vi "Rev_archivos_Calibracion.vi"() -> ()   [LabVIEW 2015]
uses:
  <vilib>/Analysis/3filter.llb/Filter Passband Type.ctl
  <vilib>/Analysis/5stat.llb/RMS (DBL).vi
  <vilib>/Analysis/baseanly.llb/Mean (DBL).vi
  <vilib>/Analysis/3filter.llb/Butterworth Filter (DBL).vi
  <vilib>/measure/madcrms.llb/Basic Averaged DC-RMS for 1 Chan.vi
  <vilib>/measure/maspectr.llb/FFT Spectrum (Mag-Phase) for 1 Chan.vi
  <vilib>/Analysis/NI_AALBase.lvlib
  <vilib>/measure/NI_MAPro.lvlib
  <vilib>/Analysis/NI_AALPro.lvlib
panel:
  out "RMS conseguido":dbl format="%0.2f"
  in  "Frecuencia de excitación\ndel patrón (Hz)":sgl=159.2
  in  "Aceleración del\npatrón (g RMS)":sgl=1.0
  out "% de desv":dbl
  in  "file (use dialog)":path
  in  "Nº del canal":i32
  out "Desviación típica":dbl format="%0.2f"
  out "Promedio":dbl format="%0.2f"
  in  "Parámetro de sensibilidad\n           (mV/g) 2":sgl=10.0
  out "Número de muestras":i32
  out "FFT de la señal":cluster{"f0":dbl, "df":dbl, "magnitude":dbl[]}(graph)
  in  "Corregir":bool
  out "DC de la señal":dbl format="%#_6e"
  out "Waveform Graph":waveform(dbl)[](graph)
  out "Max, Mín":sgl[](array[numeric])
  out "Promedio absoluto (m/s2)":dbl format="%.6e"
  out "Desviación típica absoluta (m/s2)":dbl format="%.6e"
  out "Frecuencia de excitación\nVibrómetro  (Hz)":dbl
  out "Sensibilidad corregida \n         (mV/g)":dbl
  out "Promedio absoluto corregido\n              (m/s2)":dbl format="%.4f"
  out "Desviación típica absoluta corregida\n                   (m/s2)":dbl format="%.4f"
  out "Max, Mín  corregido":sgl[](array[numeric])
  in  "Parámetro de sensibilidad\n           (mV/g)":sgl=10.0
  in  "Frecuencia de muestreo 2":dbl=50000.0
  in  "Canales a calibrar (4 o 8)":u32=4
  # "ADQ Acel"
  # "ADQ Corregida"
  # "ADQ Libre"
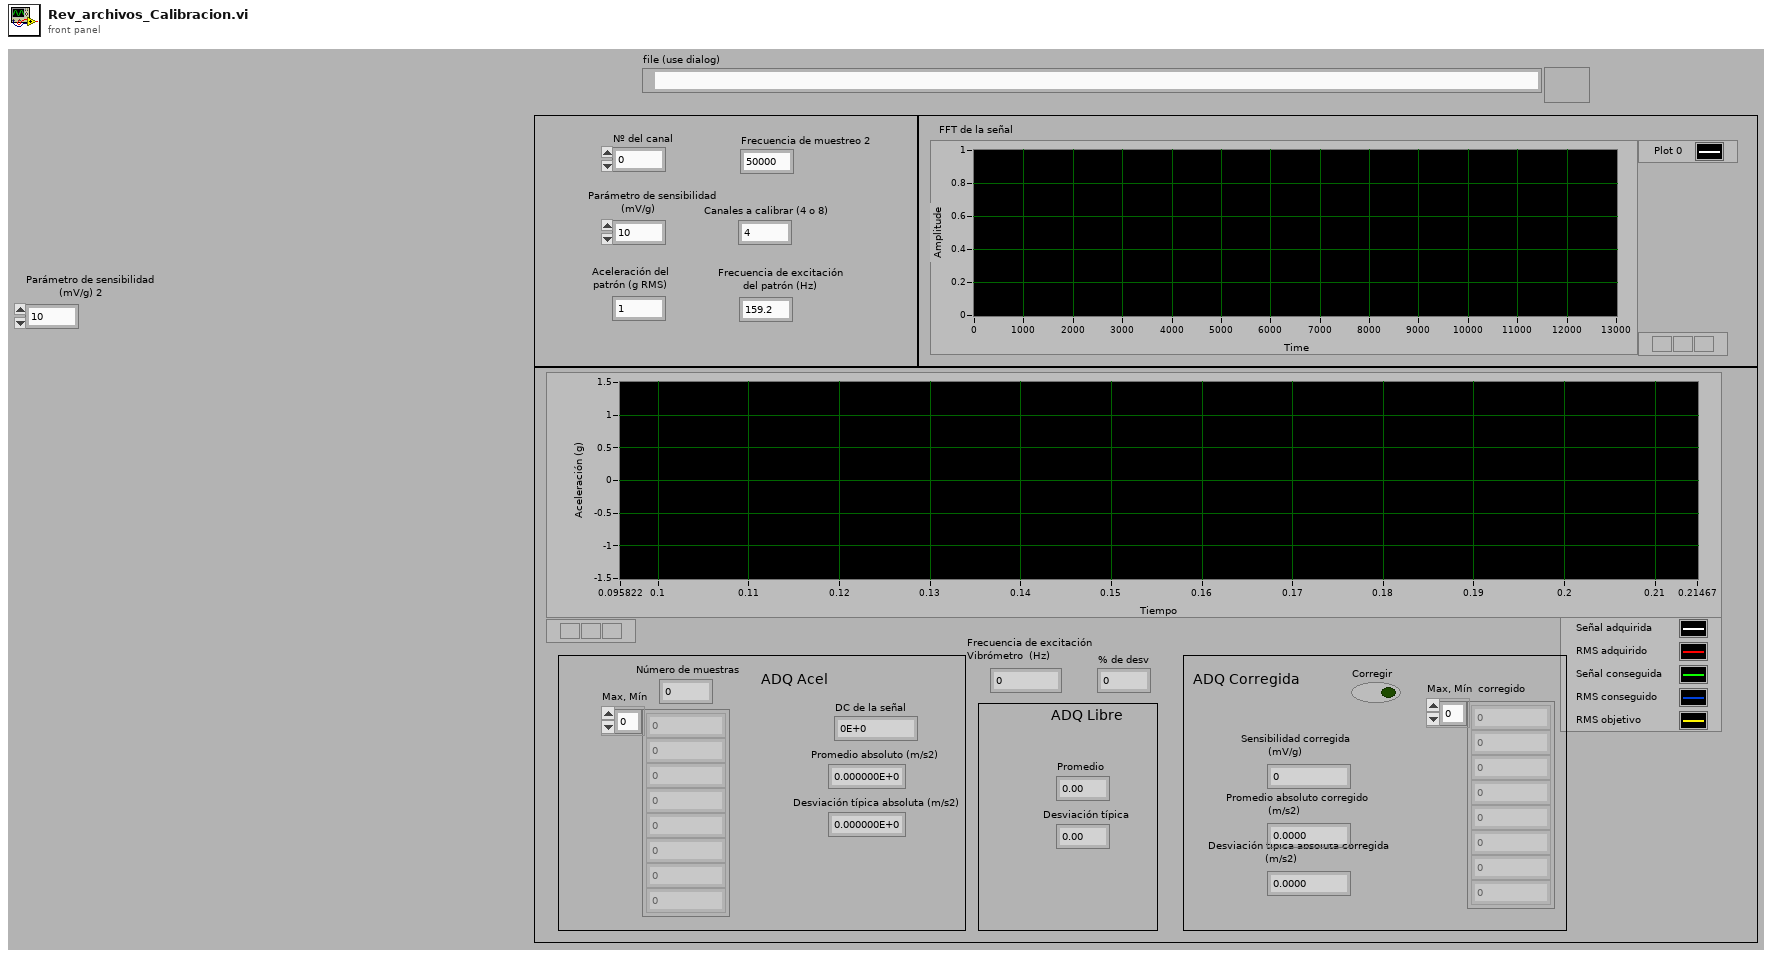
[diagram p1: front panel]
types:
  T1 = typedef "NI_AALBase.lvlib/Filter Passband Type.ctl" = enum32{"Lowpass", "Highpass", "Bandpass", "Bandstop"}
  T2 = enum16{"big-endian, network order", "native, host order", "little-endian"}
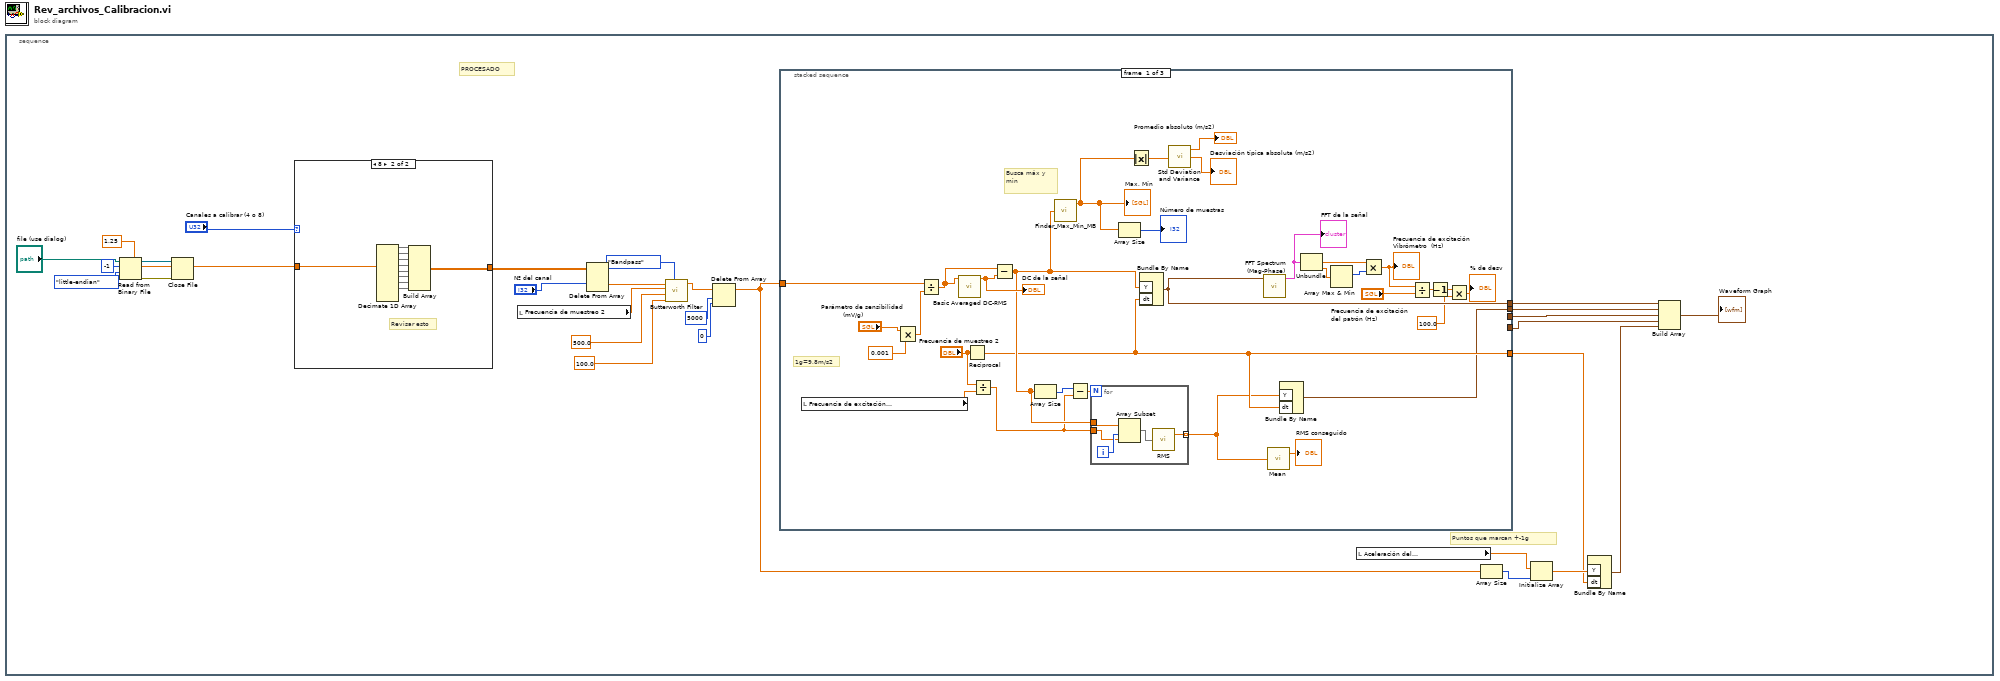
[diagram p0: block diagram]
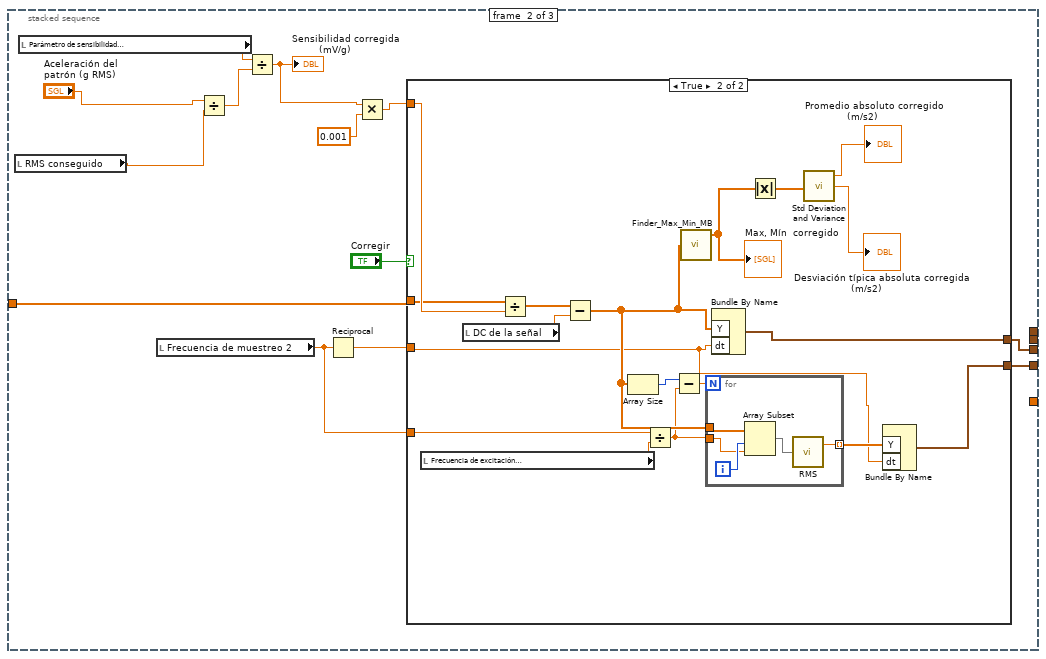
[diagram p2: hidden frame]
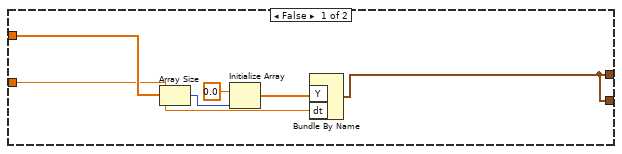
[diagram p3: hidden frame]
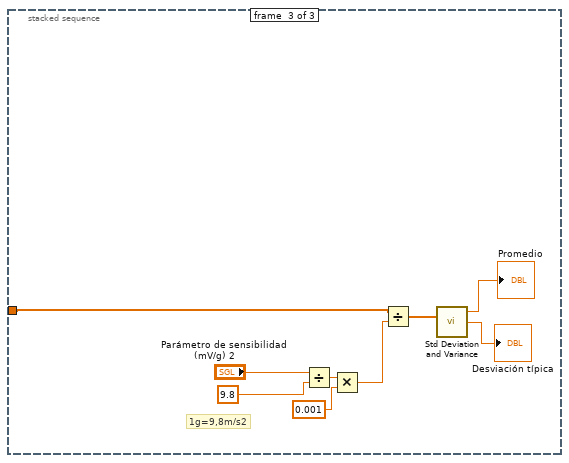
[diagram p4: hidden frame]
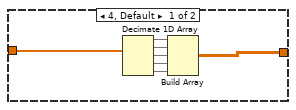
[diagram p5: hidden frame]
diagram:
  n1 = stacked-sequence {
    frame #0 {
      # "Puntos que marcan +-1g"
      # "PROCESADO"
      n2 = Read from Binary File(5:sgl 1.25, 9:T2."little-endian" ("byte order (0:big-endian, network order)"), 10:-1 ("count (1)"), 11:"file (use dialog)") -> (0:w29:errorcluster, 2:w24:sgl[], 3:w26:refnum<file>)  [unwired: 1 in, 2 out]
      n3 = Close File(refnum=w26, error in=w29) -> ()  [unwired: 2 out]
      n4 = case shown="8" "Canales a calibrar (4 o 8)" {
        tunnel: w24 -> [w121 w131]
        tunnel: [w120 w130] -> w23
        frame 4, Default {
          n5 = Decimate 1D Array(w121) -> (w123:sgl[], w124:sgl[], w122:sgl[], w119:sgl[], w118:sgl[])
          n6 = Build Array(w123, w124, w122, w119, w118) -> (w120:sgl[][])
        }
        frame 8 {
          # "Revisar esto"
          n7 = Decimate 1D Array(w131) -> (w133:sgl[], w134:sgl[], w132:sgl[], w126:sgl[], w125:sgl[], w127:sgl[], w128:sgl[], w129:sgl[])  [unwired: 2 out]
          n8 = Build Array(w133, w134, w132, w126, w125, w127, w128, w129) -> (w130:sgl[][])
        }
      }
      n9 = local read "Frecuencia de muestreo 2"() -> (w12:dbl)
      n10 = Delete From Array(array=w23, index (row)="Nº del canal") -> (deleted portion=w13:sgl[])  [unwired: 2 in, 1 out]
      n11 = call-poly <vilib>:"Butterworth Filter.vi"("filter type"=Filter_Passband_Type."Bandpass", "low cutoff freq: fl"=100.0, "high cutoff freq: fh"=500.0, "sampling freq: fs"=w12, "X"=w13) -> ("Filtered X"=w8:dbl[])  [unwired: 3 in, 1 out]
      n12 = Delete From Array(array=w8, length=5000, index=0) -> (array with subset deleted=w6:dbl[])  [unwired: 1 out]
      n13 = stacked-sequence {
        tunnel: [w53 _ _] -> w22
        tunnel: [w33 _ _] -> w19
        tunnel: w6 -> [w39 w79 w112]
        tunnel: [w32 _ _] -> w17
        tunnel: [_ w72 _] -> w4
        tunnel: [_ w71 _] -> w1
        frame #0 {
          # "Busca máx y\nmin"
          # "1g=9,8m/s2"
          n14 = local read "Frecuencia de excitación\ndel patrón (Hz)"() -> (w35:sgl)
          n15 = Multiply(x="Parámetro de sensibilidad\n           (mV/g)", y=0.001) -> (x*y=w44:dbl)
          n16 = Divide(x=w39, y=w44) -> (x/y=w38:dbl[])
          n17 = call-poly <vilib>:"Basic Averaged DC-RMS.vi"("signal in"=w38) -> ("DC value"=w50:dbl)  [unwired: 7 in, 3 out]
          "DC de la señal" <- w50
          n18 = Reciprocal(x="Frecuencia de muestreo 2") -> (1/x=w33:dbl)
          n19 = Divide(x="Frecuencia de muestreo 2", y=w35) -> (x/y=w34:dbl)
          n20 = Subtract(x=w38, y=w50) -> (x-y=w37:dbl[])
          n21 = Array Size(array=w37) -> (size(s)=w40:i32)
          n22 = call "Finder_Max_Min_MB.vi"("Señal\nAcelerómetro"=w37) -> ("Max, Mín"=w55:sgl[])  [unwired: 7 in, 1 out]
          "Max, Mín" <- w55
          n23 = Subtract(x=w40, y=w34) -> (x-y=w41:dbl)
          n24 = for {
            N: w41 -> [_]
            tunnel: w34 -> [w63]
            tunnel: [w66] -> w31 mode=indexing
            tunnel: w37 -> [w65]
            i -> [w64]
            n25 = Array Subset(array=w65, index=w64, length=w63) -> (w62:dbl[])
            n26 = call-poly <vilib>:"RMS.vi"("X"=w62) -> ("rms value"=w66:dbl)  [unwired: 1 out]
          }
          n27 = Array Size(array=w55) -> (size(s)=→"Número de muestras":i32)
          n28 = Absolute Value(x=w55) -> (abs(x)=w61:sgl[])
          n29 = Bundle By Name("Y"=w37, "dt"=w33) -> (w53:waveform(dbl))  [unwired: 1 in]
          n30 = call <vilib>:"Std Deviation and Variance.vi"("X"=w61) -> ("mean"=→"Promedio absoluto (m/s2)":dbl, "standard deviation"=→"Desviación típica absoluta (m/s2)":dbl)  [unwired: 1 in, 1 out]
          n31 = call-poly <vilib>:"FFT Spectrum (Mag-Phase).vi"("time signal"=w53) -> ("magnitude"=w57:cluster{"f0":dbl, "df":dbl, "magnitude":dbl[]})  [unwired: 6 in, 4 out]
          "FFT de la señal" <- w57
          n32 = call-poly <vilib>:"Mean.vi"("X"=w31) -> ("mean"=→"RMS conseguido":dbl)  [unwired: 1 out]
          n33 = Bundle By Name("Y"=w31, "dt"=w33) -> (w32:waveform(dbl))  [unwired: 1 in]
          n34 = Unbundle(w57) -> ("df"=w58:dbl, "magnitude"=w59:dbl[])  [unwired: 1 out]
          n35 = Array Max & Min(array=w59) -> (max index (indices)=w60:i32)  [unwired: 3 out]
          n36 = Multiply(x=w58, y=w60) -> (x*y=w49:dbl)
          "Frecuencia de excitación\nVibrómetro  (Hz)" <- w49
          n37 = Divide(x=w49, y="Frecuencia de excitación\ndel patrón (Hz)") -> (x/y=w48:dbl)
          n38 = Decrement(x=w48) -> (x-1=w47:dbl)
          n39 = Multiply(x=w47, y=100.0) -> (x*y=→"% de desv":dbl)
        }
        frame #1 {
          n40 = local read "RMS conseguido"() -> (w70:dbl)
          n41 = local read "Parámetro de sensibilidad\n           (mV/g)"() -> (w75:sgl)
          n42 = local read "Frecuencia de muestreo 2"() -> (w67:dbl)
          n43 = Divide(x="Aceleración del\npatrón (g RMS)", y=w70) -> (x/y=w77:dbl)
          n44 = Divide(x=w75, y=w77) -> (x/y=w68:dbl)
          "Sensibilidad corregida \n         (mV/g)" <- w68
          n45 = Reciprocal(x=w67) -> (1/x=w76:dbl)
          n46 = Multiply(x=w68, y=0.001) -> (x*y=w73:dbl)
          n47 = case shown="True" "Corregir" {
            tunnel: w79 -> [w82 w96]
            tunnel: w73 -> [_ w103]
            tunnel: [w80 w98] -> w72
            tunnel: w76 -> [w81 w88]
            tunnel: [w80 w87] -> w71
            tunnel: w67 -> [_ w86]
            frame False {
              n48 = Array Size(array=w82) -> (size(s)=w85:i32)
              n49 = Initialize Array(0.0 ("element"), w85) -> (w83:dbl[])
              n50 = Bundle By Name("Y"=w83, "dt"=w81) -> (w80:waveform(dbl))  [unwired: 1 in]
            }
            frame True {
              n51 = local read "Frecuencia de excitación\ndel patrón (Hz)"() -> (w91:sgl)
              n52 = local read "DC de la señal"() -> (w97:dbl)
              n53 = Divide(x=w96, y=w103) -> (x/y=w95:dbl[])
              n54 = Subtract(x=w95, y=w97) -> (x-y=w90:dbl[])
              n55 = Array Size(array=w90) -> (size(s)=w93:i32)
              n56 = Divide(x=w86, y=w91) -> (x/y=w89:dbl)
              n57 = Subtract(x=w93, y=w89) -> (x-y=w94:dbl)
              n58 = call "Finder_Max_Min_MB.vi"("Señal\nAcelerómetro"=w90) -> ("Max, Mín"=w99:sgl[])  [unwired: 7 in, 1 out]
              "Max, Mín  corregido" <- w99
              n59 = for {
                N: w94 -> [_]
                tunnel: w89 -> [w105]
                tunnel: [w108] -> w92 mode=indexing
                tunnel: w90 -> [w107]
                i -> [w106]
                n60 = Array Subset(array=w107, index=w106, length=w105) -> (w104:dbl[])
                n61 = call-poly <vilib>:"RMS.vi"("X"=w104) -> ("rms value"=w108:dbl)  [unwired: 1 out]
              }
              n62 = Bundle By Name("Y"=w90, "dt"=w88) -> (w98:waveform(dbl))  [unwired: 1 in]
              n63 = Absolute Value(x=w99) -> (abs(x)=w102:sgl[])
              n64 = call <vilib>:"Std Deviation and Variance.vi"("X"=w102) -> ("mean"=→"Promedio absoluto corregido\n              (m/s2)":dbl, "standard deviation"=→"Desviación típica absoluta corregida\n                   (m/s2)":dbl)  [unwired: 1 in, 1 out]
              n65 = Bundle By Name("Y"=w92, "dt"=w88) -> (w87:waveform(dbl))  [unwired: 1 in]
            }
          }
        }
        frame #2 {
          # "1g=9,8m/s2"
          n66 = Divide(x="Parámetro de sensibilidad\n           (mV/g) 2", y=9.8) -> (x/y=w115:dbl)
          n67 = Multiply(x=w115, y=0.001) -> (x*y=w114:dbl)
          n68 = Divide(x=w112, y=w114) -> (x/y=w109:dbl[])
          n69 = call <vilib>:"Std Deviation and Variance.vi"("X"=w109) -> ("mean"=→"Promedio":dbl, "standard deviation"=→"Desviación típica":dbl)  [unwired: 1 in, 1 out]
        }
      }
      n70 = local read "Aceleración del\npatrón (g RMS)"() -> (w3:sgl)
      n71 = Array Size(array=w6) -> (size(s)=w21:i32)
      n72 = Initialize Array(w3, w21) -> (w20:sgl[])
      n73 = Bundle By Name("Y"=w20, "dt"=w19) -> (w2:waveform(sgl))  [unwired: 1 in]
      n74 = Build Array(w22, w17, w4, w1, w2) -> (→"Waveform Graph":waveform(dbl)[])
    }
  }
